vi "POV up or downish.vi"(10 "POV":i16[](array[numeric])) -> (1 "DOWNish":bool, 2 "UPish":bool)   [LabVIEW 2017]
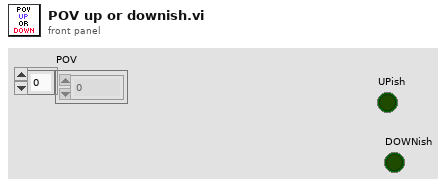
[diagram p1: front panel]
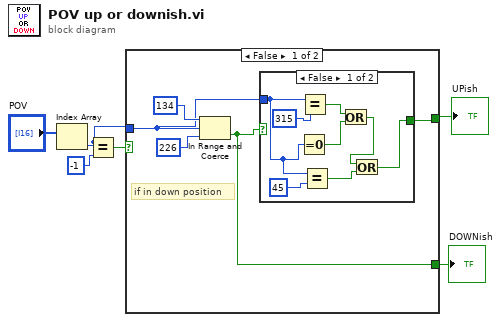
[diagram p0: block diagram]
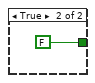
[diagram p2: hidden frame]
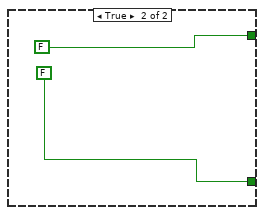
[diagram p3: hidden frame]
diagram:
  n1 = Index Array(array="POV") -> (element=w1:i16)  [unwired: 1 in]
  n2 = Equal?(x=w1, y=i16 -1) -> (x = y?=w5:bool)
  n3 = case shown="False" w5 {
    tunnel: [w9 FALSE] -> w3
    tunnel: [w7 FALSE] -> w2
    tunnel: w1 -> [w8 _]
    frame False {
      # "if in down position"
      n4 = In Range and Coerce(upper limit=i16 134, x=w8, lower limit=i16 226) -> (In Range?=w7:bool)  [unwired: 1 out]
      n5 = case shown="False" w7 {
        tunnel: [w12 FALSE] -> w9
        tunnel: w8 -> [w18 _]
        frame False {
          n6 = Equal To 0?(x=w18) -> (x = 0?=w15:bool)
          n7 = Equal?(x=w18, y=i16 315) -> (x = y?=w16:bool)
          n8 = Equal?(x=w18, y=i16 45) -> (x = y?=w13:bool)
          n9 = Or(x=w16, y=w15) -> (x .or. y?=w14:bool)
          n10 = Or(x=w14, y=w13) -> (x .or. y?=w12:bool)
        }
        frame True {
        }
      }
    }
    frame True {
    }
  }
  "UPish" <- w3
  "DOWNish" <- w2
